vi "Determine Page Title.vi"(7 "Update Current Page (F)":bool, 8 "error in (no error)":errorcluster {"code" format="Error %.0f"}, 10 "Name":string, 11 "VIDoc Printer - Confluence In":refnum<class "VIDoc Printer - Confluence.lvclass">) -> (0 "error out":errorcluster {"code" format="Error %.0f"}, 1 "Parent Page Title":string, 2 "Page Title":string, 3 "VIDoc Printer - Confluence Out":refnum<class "VIDoc Printer - Confluence.lvclass">)   [LabVIEW 2023, in "VIDoc Printer - Confluence.lvlib" / "VIDoc Printer - Confluence.lvclass"]
uses:
  VIDoc Printer - Confluence.lvclass
  VIDoc Printer - Confluence.lvclass/VIDoc Printer - Confluence.ctl
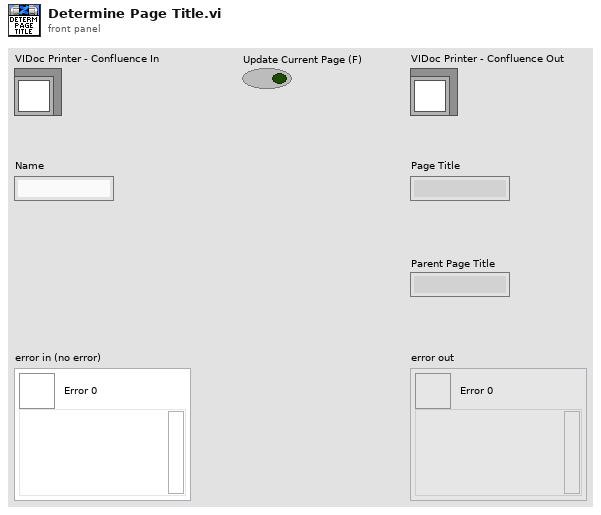
[diagram p1: front panel]
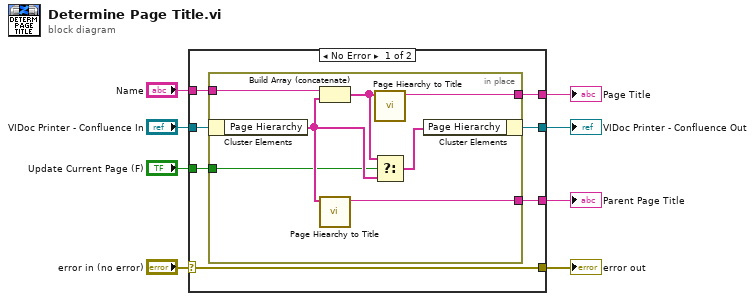
[diagram p0: block diagram]
diagram:
  n1 = case shown="No Error" "error in (no error)" {
    selector: "error in (no error)" -> [w15 w24]
    tunnel: [w15 w24] -> w7
    tunnel: [w13 w23] -> w5
    tunnel: "VIDoc Printer - Confluence In" -> [w14 w23]
    tunnel: "Name" -> [w12 _]
    tunnel: "Update Current Page (F)" -> [w11 _]
    tunnel: [w10 _] -> w2
    tunnel: [w9 _] -> w1
    frame No Error {
      n2 = in-place {
        in-place-border: w12 -> [w22]
        in-place-border: w11 -> [w18]
        in-place-border: [w17] -> w10
        in-place-border: [w16] -> w9
        n3 = in-place-cluster #1(w14) -> ("Page Hierarchy"=w19:string[])
        n4 = Build Array (concatenate)(w22, w19) -> (w21:string[])
        n5 = call "Page Hiearchy to Title.vi"("Page Hierarchy"=w19) -> ("Page Title"=w16:string)  [unwired: 10 in]
        n6 = call "Page Hiearchy to Title.vi"("Page Hierarchy"=w21) -> ("Page Title"=w17:string)  [unwired: 10 in]
        n7 = Select(t=w21, s=w18, f=w19) -> (s? t:f=w20:string[])
        n8 = in-place-cluster #1("Page Hierarchy"=w20) -> (w13:refnum<class "VIDoc Printer - Confluence.lvclass">)
      }
    }
    frame Error {
    }
  }
  "error out" <- w7
  "VIDoc Printer - Confluence Out" <- w5
  "Page Title" <- w2
  "Parent Page Title" <- w1
